vi "SetBounds.vi"(8 "error in (no error)":errorcluster, 10 "bounds":cluster{"width":u32, "height":u32}, 11 "text in":refnum<class "text.lvclass">) -> (0 "error out":errorcluster, 3 "text out":refnum<class "text.lvclass">)   [LabVIEW 2009, in "text.lvclass"]
uses:
  text.lvclass
  text.lvclass/text.ctl
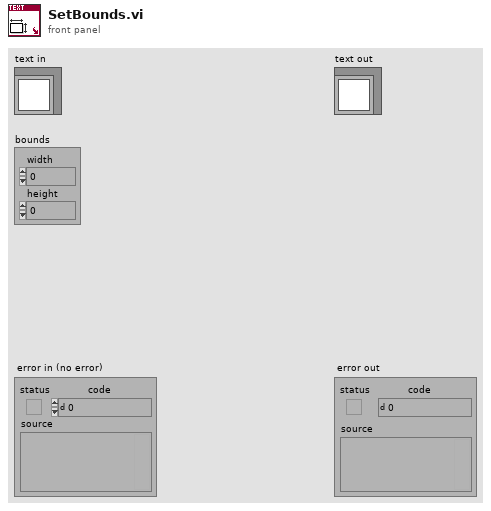
[diagram p1: front panel]
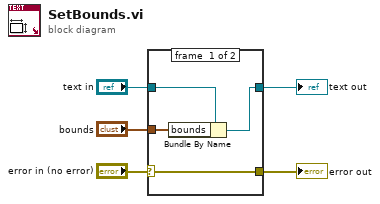
[diagram p0: block diagram]
diagram:
  n1 = case shown="No Error" "error in (no error)" {
    selector: "error in (no error)" -> [w8 w11]
    tunnel: [w8 w11] -> w2
    tunnel: [w7 w10] -> w4
    tunnel: "text in" -> [w9 w10]
    tunnel: "bounds" -> [w6 _]
    frame #0 {
      n2 = Bundle By Name(cluster=w9, "bounds"=w6) -> (w7:refnum<class "text.lvclass">)
    }
    frame #1 {
    }
  }
  "text out" <- w4
  "error out" <- w2
